vi "Write Flow Control Valve DAC.vi"(10 "IILCDAC":refnum<class "IILCDAC.lvclass">, 11 "ILCControlledActuatorCylinder in":refnum<class "ILCControlledActuatorCylinder.lvclass">) -> (3 "ILCControlledActuatorCylinder out":refnum<class "ILCControlledActuatorCylinder.lvclass">)   [LabVIEW 2015, in "ILCControlledActuatorCylinder.lvclass"]
uses:
  ILCControlledActuatorCylinder.lvclass
  ILCDAC/IILCDAC/IILCDAC.lvclass
  ILCControlledActuatorCylinder.lvclass/ILCControlledActuatorCylinder.ctl
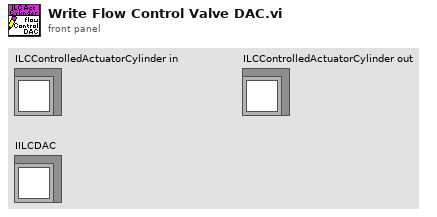
[diagram p1: front panel]
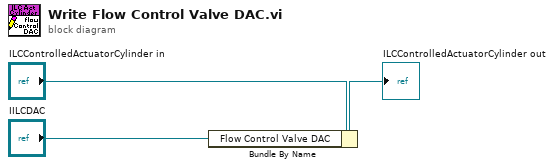
[diagram p0: block diagram]
diagram:
  n1 = Bundle By Name(cluster="ILCControlledActuatorCylinder in", "Flow Control Valve DAC"="IILCDAC") -> (→"ILCControlledActuatorCylinder out":refnum<class "ILCControlledActuatorCylinder.lvclass">)
